vi "Abort Move SubVi.vi"(2 "error in":errorcluster, 3 "reference in":refnum<k24>) -> (0 "error out":errorcluster, 1 "reference out":refnum<k24>)   [LabVIEW 2017]
uses:
  Newport.XPS.CommandInterface
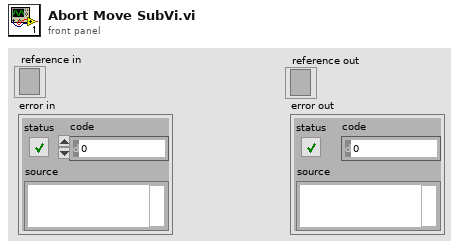
[diagram p1: front panel]
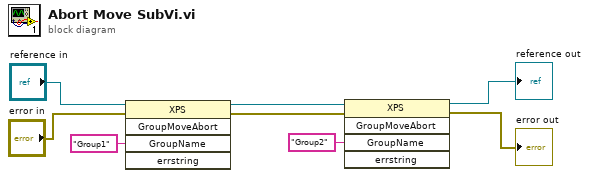
[diagram p0: block diagram]
diagram:
  n1 = invoke class="XPS" method="GroupMoveAbort"(reference="reference in", error in="error in", "GroupName"="Group1") -> (reference out=w2:refnum<k24>, error out=w1:errorcluster)  [unwired: 2 in, 3 out]
  n2 = invoke class="XPS" method="GroupMoveAbort"(reference=w2, error in=w1, "GroupName"="Group2") -> (reference out=→"reference out":refnum<k24>, error out=→"error out":errorcluster)  [unwired: 2 in, 3 out]
